vi "SensorTest.vi"() -> ()   [LabVIEW 2012]
uses:
  <vilib>/FPGAPlugInAG/sbRIO-9642/niLvFpga_Open_sbRIO-9642.vi
  <vilib>/rvi/interface/common/dynamic/niFpgaDynamicAddResources.vi
  <vilib>/Utility/error.llb/Error Cluster From Error Code.vi
  <vilib>/rvi/errors/niLvFpgaAdjustHostInterfaceError.vi
  <vilib>/rvi/interface/nirviOpenFPGA/nirviOpenFPGA.xnode
  My Documents/ARTV/FPGA Bitfiles/SensorFusion_FPGATarget_IRInputKevin_bDJ353ADX2A.lvbitx
  My Documents/ARTV/IR_Input_Kevin.vi
  <vilib>/rvi/interface/nirviReadWriteControl/nirviReadWriteControl.xnode
  <vilib>/robotics/Starter Kit/Host Interface/NI_Robotics_Starter Kit Host.lvclass
  NiFpgaLv.dll
  <vilib>/rvi/interface/Simulation/niFpgaSimulationCallBeginRW.vi
panel:
  in  "IMU Request":i32(listbox) caption="Listbox"
  out "Sensor Data":T1={"Left Distance Sensors"={"IR"=0.0, "Sonar"=0.0, "Fusion"=0.0}, "Right Distance Sensors"={"IR"=0.0, "Sonar"=0.0, "Fusion"=0.0}, "IMU Data"={"gyro x"=0.0, "gyro y"=0.0610352, "gyro z"=0.0610352, "acc x "=0.015930135, "acc y"=-0.056945655, "acc z"=-1.04699439, "mag x"=-1.516114368, "mag y"=0.941773136, "mag z"=2.677614224, "euler phi"=0.29663009999999995, "euler theta"=9.722875499999999, "euler psi"=-67.3240464}} {"Right Distance Sensors"."Fusion" scale=0.0..200.0 scale format="%#.2f"; "Right Distance Sensors"."Sonar" scale=0.0..200.0 scale format="%#.2f"; "Right Distance Sensors"."IR" scale=0.0..200.0 scale format="%#.2f"; "Left Distance Sensors"."Fusion" scale=0.0..200.0 scale format="%#.2f"; "Left Distance Sensors"."Sonar" scale=0.0..200.0 scale format="%#.2f"; "Left Distance Sensors"."IR" scale=0.0..200.0 scale format="%#.2f"}
  out "Distance Sensor Data":dbl[][](array[slide]) scale=0.0..200.0
  in  "ModA/AI3 2":fxp<+/-,26,5>
  in  "ModA/AI2 2":fxp<+/-,26,5>
  in  "ModA/AI1 2":fxp<+/-,26,5>
  in  "ModA/AI0 2":fxp<+/-,26,5>
  out "Sonar\nDistance Display":dbl[](array[slide]) scale=0.0..200.0
  out "IR Distance Display":dbl[](array[slide]) scale=0.0..200.0
  out "ModA/AI3":fxp<+/-,26,5>
  out "Sonar\nAnalog Values":fxp<+/-,26,5>[](array[numeric])
  out "Sonar\nDistance":dbl[](array[numeric]) format="%0.2f"
  out "ModA/AI2":fxp<+/-,26,5>
  out "IR Analog Values":fxp<+/-,26,5>[](array[numeric])
  out "IR Distance":dbl[](array[numeric]) format="%0.2f"
  out "interpolation value":dbl format="%0.2f"
  in  "sampling freq: fs":dbl=20.0 format="%0.2f"
  in  "low cutoff freq: fl":dbl=5.0 format="%0.4f"
  in  "order":i32=1
  out "ModA/AI0_orig":fxp<+/-,26,5>=-4.425695419311523 format="%.3g"
  in  "stop":bool
  out "ModA/AI1":fxp<+/-,26,5>
  out "ModA/AI0":fxp<+/-,26,5>
  # "Unused/Commented Out"
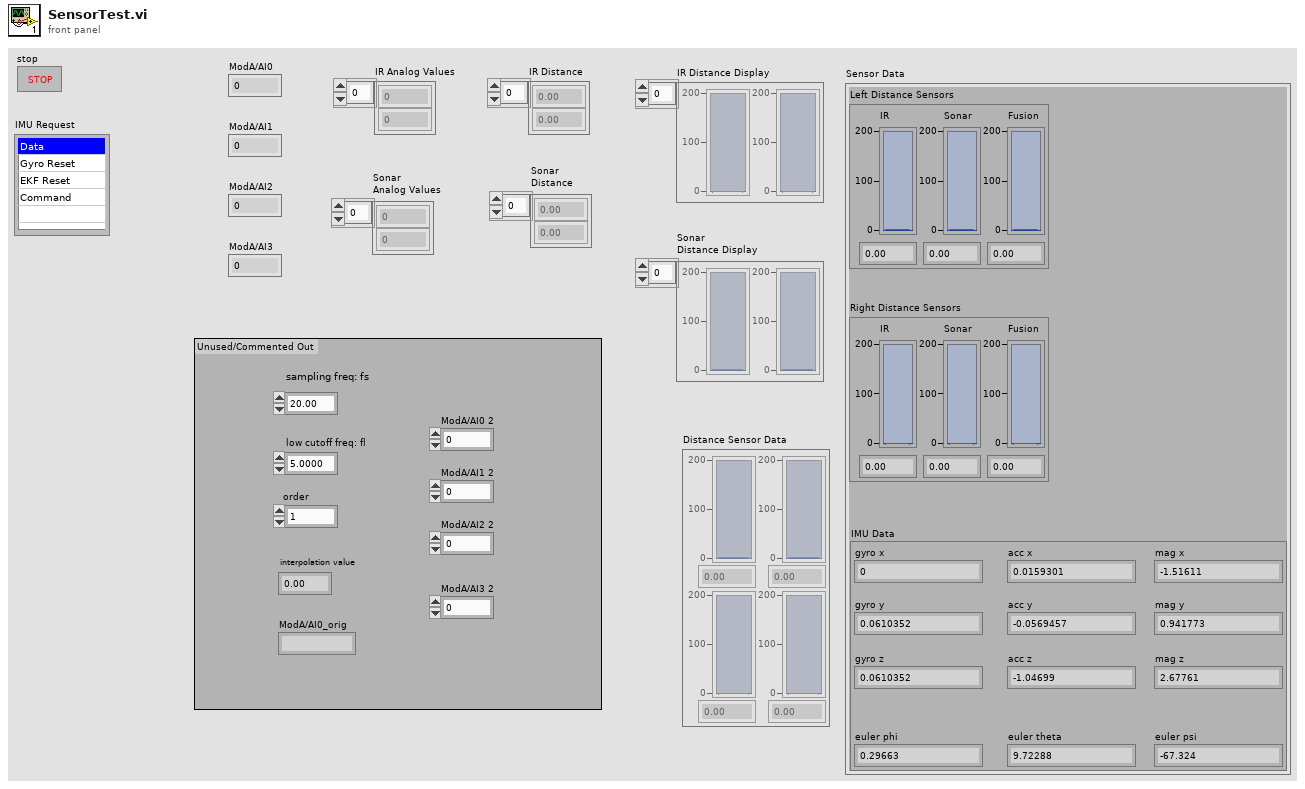
[diagram p1: front panel]
types:
  T1 = cluster{"Left Distance Sensors":cluster{"IR":dbl, "Sonar":dbl, "Fusion":dbl}, "Right Distance Sensors":cluster{"IR":dbl, "Sonar":dbl, "Fusion":dbl}, "IMU Data":cluster{"gyro x":dbl, "gyro y":dbl, "gyro z":dbl, "acc x ":dbl, "acc y":dbl, "acc z":dbl, "mag x":dbl, "mag y":dbl, "mag z":dbl, "euler phi":dbl, "euler theta":dbl, "euler psi":dbl}}
  T2 = cluster{"gyro x":dbl, "gyro y":dbl, "gyro z":dbl, "acc x ":dbl, "acc y":dbl, "acc z":dbl, "mag x":dbl, "mag y":dbl, "mag z":dbl, "euler phi":dbl, "euler theta":dbl, "euler psi":dbl}
  T3 = cluster{"[0]":cluster{"interpolation value":dbl, dbl, dbl}, "[1]":cluster{"interpolation value":dbl, dbl, dbl}}
  T4 = cluster{"[0]":cluster{"interpolation value":dbl, dbl, dbl}, "[1]":cluster{"interpolation value":dbl, dbl, dbl}, "IMU Data":cluster{"gyro x":dbl, "gyro y":dbl, "gyro z":dbl, "acc x ":dbl, "acc y":dbl, "acc z":dbl, "mag x":dbl, "mag y":dbl, "mag z":dbl, "euler phi":dbl, "euler theta":dbl, "euler psi":dbl}}
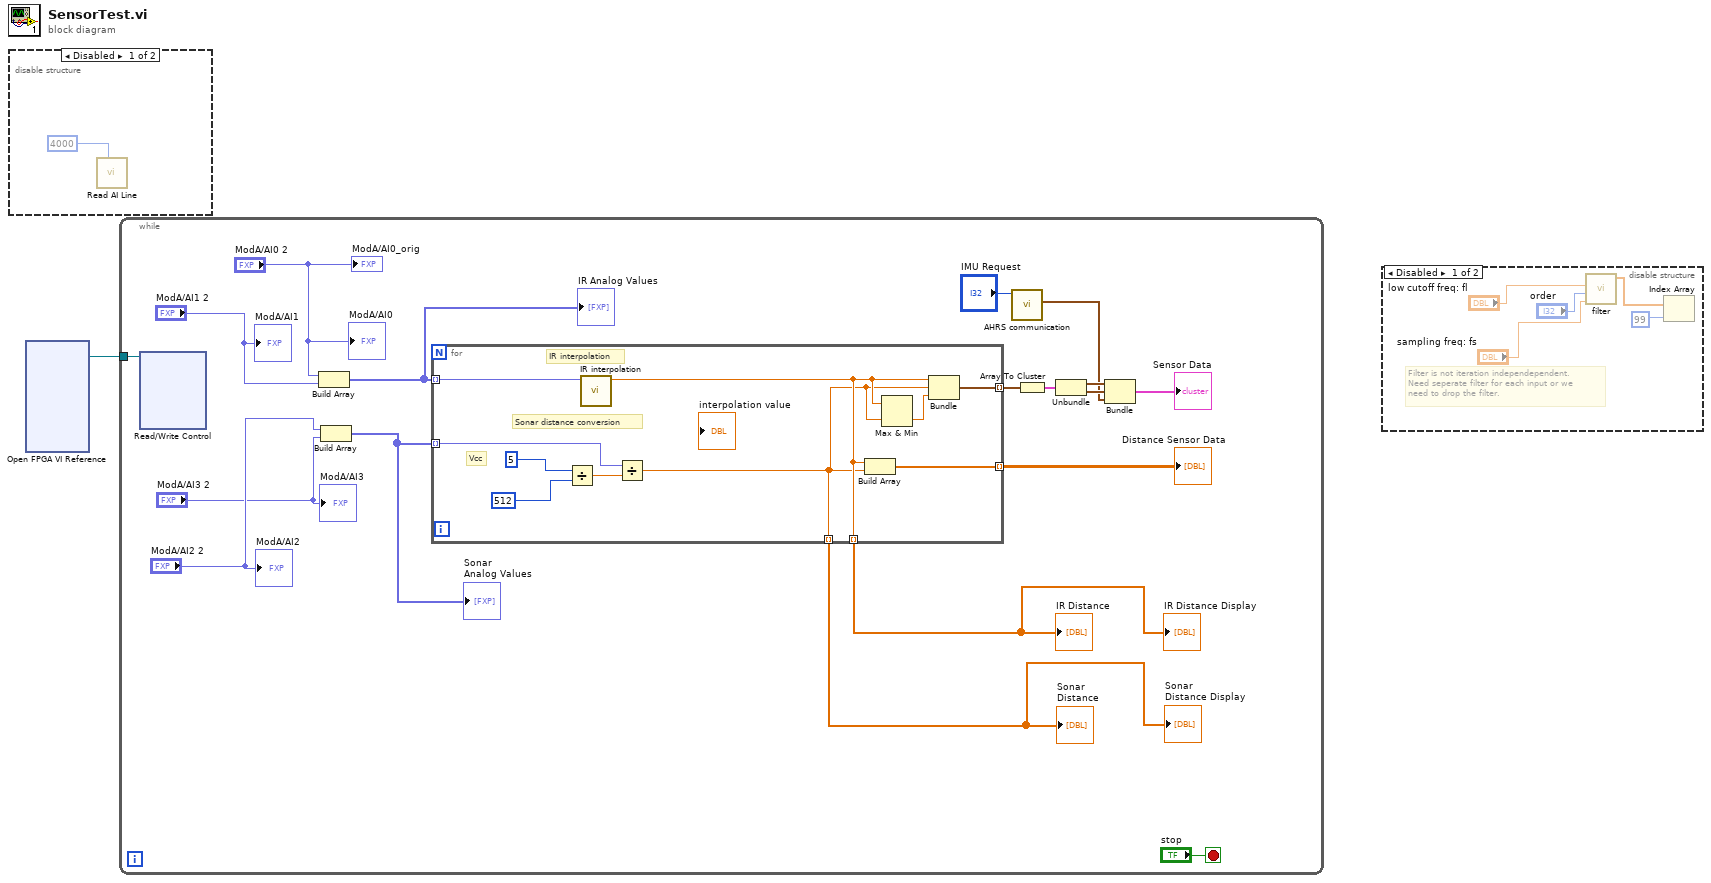
[diagram p0: block diagram]
diagram:
  n1 = disable-structure shown="Disabled" {
    frame Disabled {
      n2 = call <vilib>:"Read AI Line.vi"("AI line"=4000 ("low cutoff freq: fl")) -> ()  [unwired: 8 in, 3 out]
    }
    frame Enabled {
    }
  }
  n3 = xnode "Open FPGA VI Reference"() -> ("FPGA VI Reference Out"=w1:refnum<k20>)  [unwired: 2 in, 1 out]
  n4 = while {
    tunnel: w1 -> [w19]
    stop <- "stop" stop-if-true
    n5 = xnode "Read/Write Control"("FPGA VI Reference In"=w19) -> ()  [unwired: 1 in, 6 out]
    n6 = Build Array("ModA/AI0 2", "ModA/AI1 2") -> (w13:fxp<+/-,26,5>[])
    "IR Analog Values" <- w13
    n7 = Build Array("ModA/AI2 2", "ModA/AI3 2") -> (w14:fxp<+/-,26,5>[])
    "Sonar\nAnalog Values" <- w14
    n8 = for {
      tunnel: w13 -> [w30] mode=indexing
      tunnel: w14 -> [w26] mode=indexing
      tunnel: [w25] -> w12 mode=indexing
      tunnel: [w24] -> w11 mode=indexing
      tunnel: [w21] -> w9 mode=indexing
      tunnel: [w22] -> w10 mode=indexing
      # "Vcc"
      # "IR interpolation"
      # "Sonar distance conversion"
      n9 = Divide(x=5, y=512) -> (x/y=w29:dbl)
      n10 = call "IR interpolation.vi"("x value"=w30) -> ("interpolation value"=w22:dbl)  [unwired: 10 in]
      n11 = Divide(x=w26, y=w29) -> (x/y=w21:dbl)
      n12 = Build Array(w22, w21) -> (w25:dbl[])
      n13 = Max & Min(x=w22, y=w21) -> (min(x,y)=w23:dbl)  [unwired: 1 out]
      n14 = Bundle("interpolation value"=w22, w21, w23) -> (w24:cluster{"interpolation value":dbl, dbl, dbl})  [unwired: 1 in]
    }
    "IR Distance" <- w10
    "Sonar\nDistance" <- w9
    "IR Distance Display" <- w10
    "Sonar\nDistance Display" <- w9
    "Distance Sensor Data" <- w12
    n15 = call "AHRS communication.vi"("Listbox"="IMU Request") -> ("IMU Data"=w4:T2)  [unwired: 10 in]
    n16 = Array To Cluster(array=w11) -> (cluster=w6:T3)
    n17 = Unbundle(w6) -> ("[0]"=w7:cluster{"interpolation value":dbl, dbl, dbl}, "[1]"=w5:cluster{"interpolation value":dbl, dbl, dbl})
    n18 = Bundle("[0]"=w7, "[1]"=w5, "IMU Data"=w4) -> (→"Sensor Data":T4)  [unwired: 1 in]
    "ModA/AI0" <- "ModA/AI0 2"
    "ModA/AI1" <- "ModA/AI1 2"
    "ModA/AI0_orig" <- "ModA/AI0 2"
    "ModA/AI2" <- "ModA/AI2 2"
    "ModA/AI3" <- "ModA/AI3 2"
  }
  n19 = disable-structure shown="Disabled" {
    frame Disabled {
      # "Filter is not iteration independependent.\nNeed seperate filter for each input or we\nneed to drop the filter."
      n20 = call "filter.vi"("sampling freq: fs"="sampling freq: fs", "order"="order", "low cutoff freq: fl"="low cutoff freq: fl") -> ("Filtered X"=w31:dbl[])  [unwired: 6 in, 2 out]
      n21 = Index Array(array=w31, index=99) -> ()  [unwired: 1 out]
    }
    frame Enabled {
    }
  }
